vi "SMBus Process Call.vi"(0 "DevType":i32, 1 "CommandCode":u8, 2 "PEC":u8, 5 "DevIndex":i32, 7 "SMBUSIndex":i32, 9 "SlaveAddr":u8, 11 "error in (no error)":errorcluster, 12 "WriteData":u16) -> (4 "pReadData":u16, 6 "function return":i32, 15 "error out":errorcluster)   [LabVIEW 2012, in "ControlSMBus.lvlib"]
doc: "int WINAPI SMBus_ProcessCall(int DevType,int DevIndex,int SMBUSIndex,unsigned char SlaveAddr,unsigned char CommandCode,unsigned short WriteData, unsigned short *pReadData,unsigned char PEC);"
uses:
  ControlSMBus.lvlib
  Ginkgo_Driver.dll
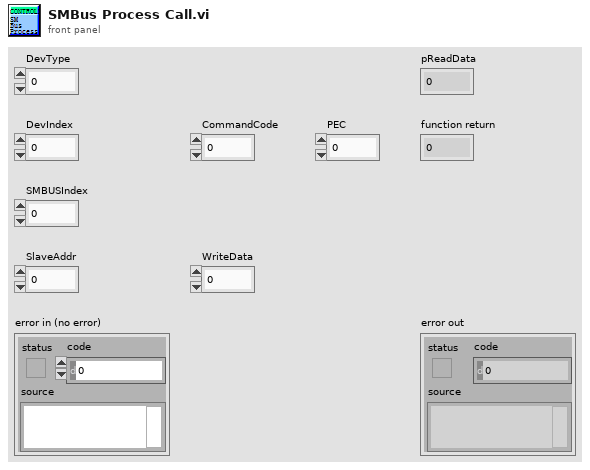
[diagram p1: front panel]
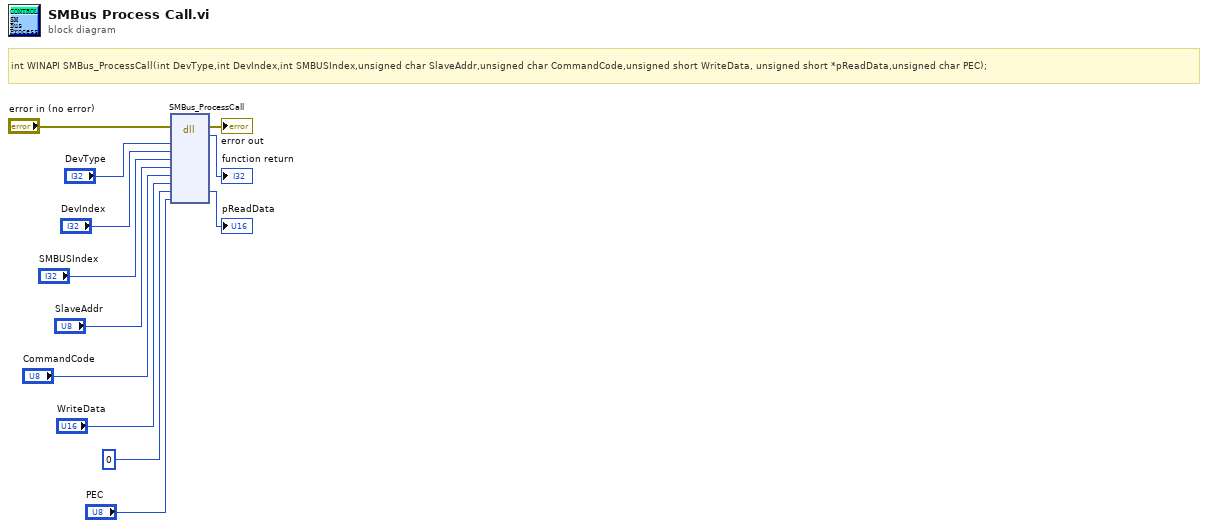
[diagram p0: block diagram]
diagram:
  # "int WINAPI SMBus_ProcessCall(int DevType,int DevIndex,int SMBUSIndex,unsigned char SlaveAddr,unsigned char CommandCode,unsigned short WriteData, unsigned short *pReadData,unsigned char PEC);"
  n1 = dll-call lib="E:/Project/vt_ginkgo/truck/Ginkgo Driver/vs2010/Ginkgo_USB-I2C_API_v2.0.3.0/lib/labview_32bit/ControlSMBus/Ginkgo_Driver.*" fn="SMBus_ProcessCall"(error in="error in (no error)", "DevType"="DevType", "DevIndex"="DevIndex", "SMBUSIndex"="SMBUSIndex", "SlaveAddr"="SlaveAddr", "CommandCode"="CommandCode", "WriteData"="WriteData", "pReadData"=u16 0, "PEC"="PEC") -> (error out=→"error out":errorcluster, →"function return":i32, "pReadData"=→"pReadData":u16)  [unwired: 9 in, 1 out]
